vi "unpackPowerState.vi"(6 "长度":i32, 7 "数据":u8[](array[numeric]) format="%.0x") -> (2 "输出通道":u8, 3 "有效状态":u8)   [LabVIEW 2014]
panel:
  out "告警信息":string
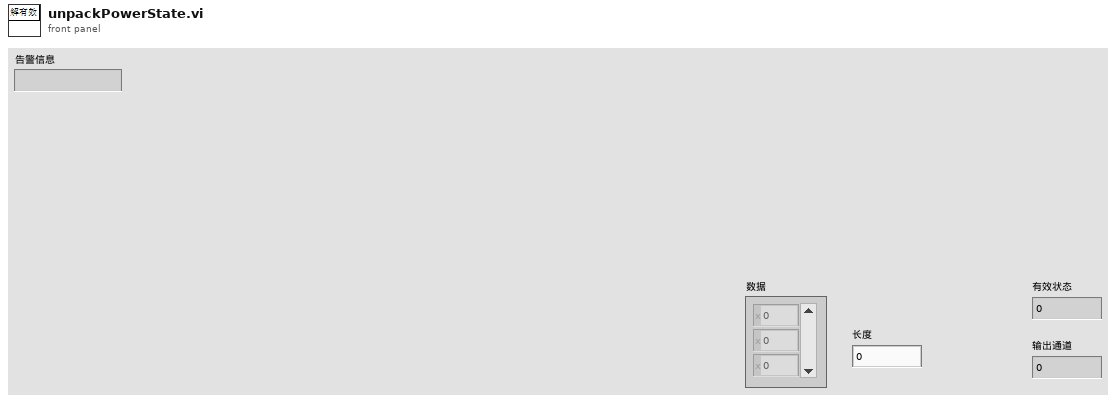
[diagram p1: front panel]
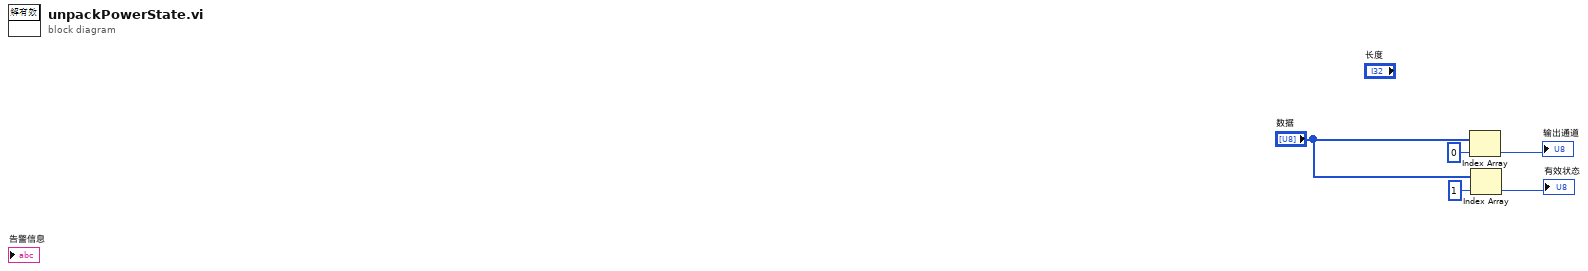
[diagram p0: block diagram]
diagram:
  n1 = Index Array(array="数据", index=0 ("索引")) -> (element=→"输出通道":u8)
  n2 = Index Array(array="数据", index=1 ("索引")) -> (element=→"有效状态":u8)
